vi "Create part number list.vi"() -> ()   [LabVIEW 2025]
panel:
  in  "Ring":u16(ring) items=["AC-97", "EVI-79-param", "EVI-79"]
  out "Array":string[](array[string])
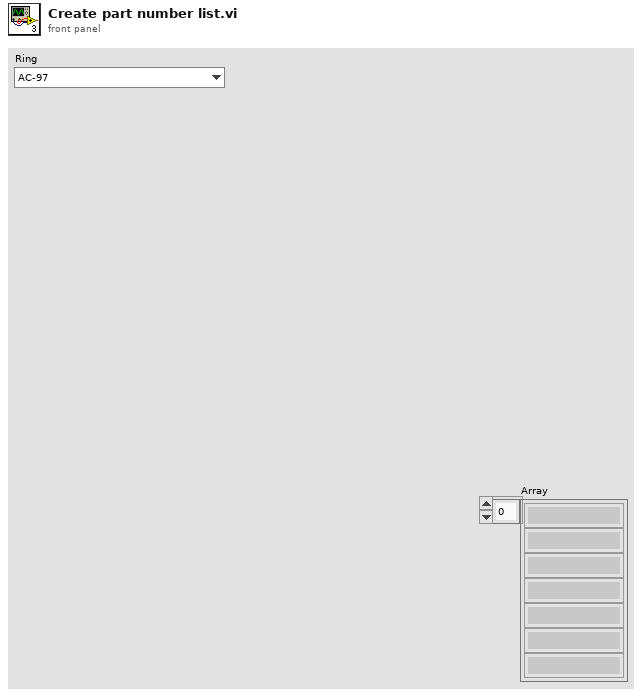
[diagram p1: front panel]
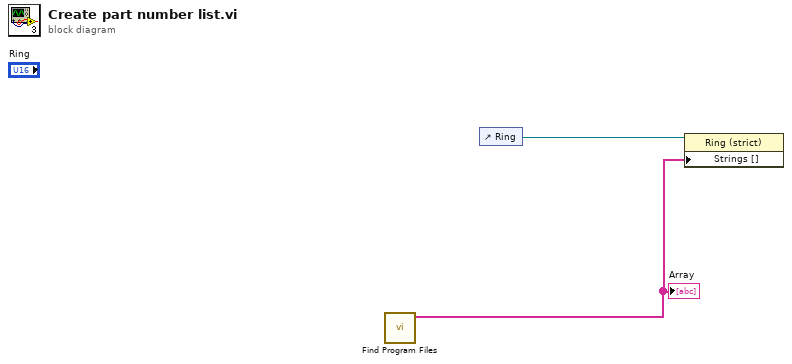
[diagram p0: block diagram]
diagram:
  n1 = call "Find Program Files.vi"() -> ("Array"=w1:string[])  [unwired: 10 in, 1 out]
  "Array" <- w1
  n2 = control-ref of="Ring"() -> (w2:refnum<vi>)
  n3 = property class="Ring (strict)"(reference=w2, "Strings []"=w1) -> ()  [unwired: 1 in, 2 out]
